vi "BotSpeak_GetVar.vi"(2 "Variable In":string="power", 3 "Bot Settings":T1) -> (0 "value":string, 1 "Bot Settings out":T1)   [LabVIEW 2012]
doc: "Retrieves the value of \"Variable in\" and returns that as \"value\". If the value is a number, this VI also returns that value in double format as \"number\"."
uses:
  <userlib>/BotSpeak/VIs/Direct/BotSpeak_Control.ctl
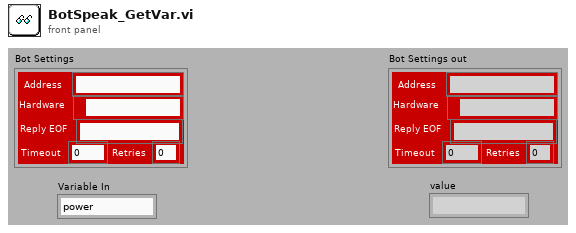
[diagram p1: front panel]
types:
  T1 = typedef "BotSpeak_Control.ctl" = cluster{"Address":string, "Reply EOF":string, "Hardware":path, "Retries":i8, "Timeout":i32}
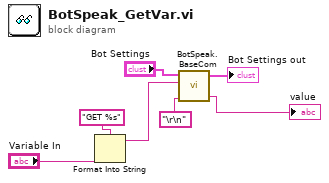
[diagram p0: block diagram]
diagram:
  n1 = Format Into String(format string="GET %s" ("command"), "Variable In") -> (resulting string=w7:string)  [unwired: 2 in, 1 out]
  n2 = call <userlib>:"BotSpeak.BaseCom.vi"("Termination"="\r\n", "command"=w7, "Bot Settings in"="Bot Settings") -> ("response"=→"value":string, "Bot Settings out"=→"Bot Settings out":T1)  [unwired: 2 in]
